vi "BrokenVI.vi"   [LabVIEW 2014]
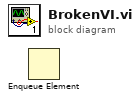
[diagram p0: block diagram]
diagram:
  n1 = Enqueue Element() -> ()  [unwired: 4 in, 3 out]
